vi "average_column_of_rand_matrix.vi"() -> ()   [LabVIEW 2021]
uses:
  <vilib>/Analysis/Matrix/Datatypes/RealMatrix.ctl
  <vilib>/Analysis/Matrix/Numeric/Conversions/Array To Matrix - RA2.vi
  <vilib>/Analysis/Matrix/NI_Matrix.lvlib
panel:
  out "sink array":dbl[][](array[numeric])
  out "sink mat":T1
  out "output":dbl[][](array[numeric])
  in  "loops":dbl
  in  "col index":dbl
  in  "blank":dbl[](array[numeric])
  out "avg":dbl
  out "num":dbl
  out "sum":dbl
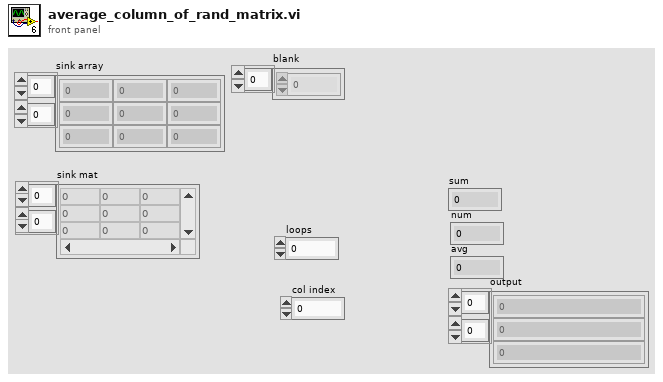
[diagram p1: front panel]
types:
  T1 = typedef "NI_Matrix.lvlib/RealMatrix.ctl" = dbl[][]
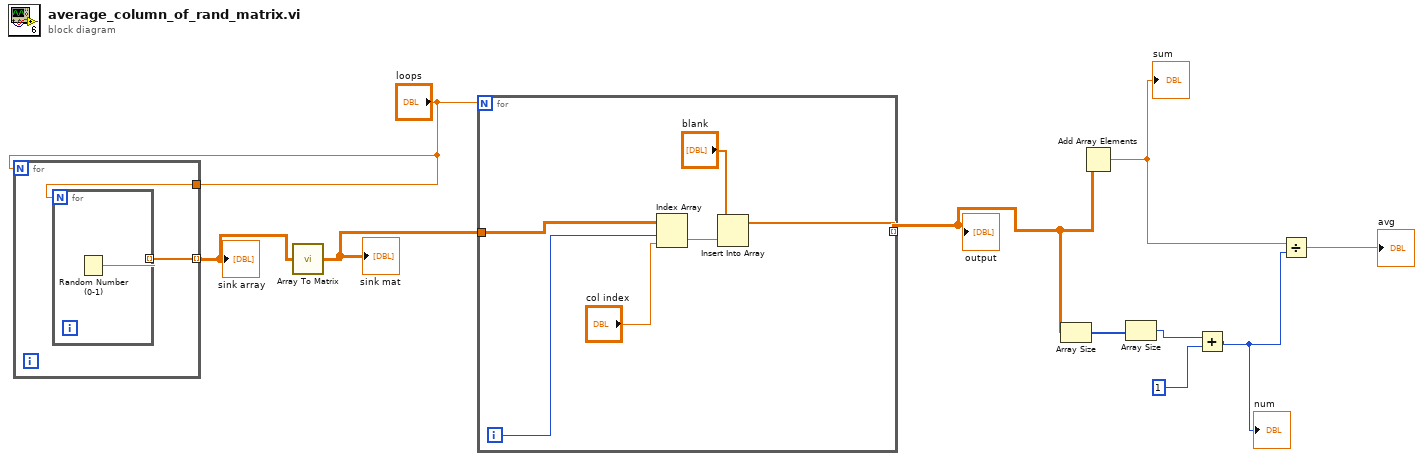
[diagram p0: block diagram]
diagram:
  n1 = for {
    N: "loops" -> [_]
    tunnel: [w12] -> w2 mode=indexing
    tunnel: "loops" -> [w11]
    n2 = for {
      N: w11 -> [_]
      tunnel: [w13] -> w12 mode=indexing
      n3 = Random Number (0-1)() -> (number: 0 to 1=w13:dbl)
    }
  }
  "sink array" <- w2
  n4 = call-poly <vilib>:"Array To Matrix.vi"("Real 2D Array"=w2) -> ("Real Matrix"=w1:T1)
  "sink mat" <- w1
  n5 = for {
    N: "loops" -> [_]
    tunnel: [w15] -> w8 mode=indexing
    tunnel: w1 -> [w14]
    i -> [w16]
    n6 = Index Array(array=w14, index (row)=w16, index (col)="col index") -> (element=w18:dbl)
    n7 = Insert Into Array(array="blank", new element=w18) -> (w15:dbl[])  [unwired: 1 in]
  }
  "output" <- w8
  n8 = Array Size(array=w8) -> (size(s)=w7:i32[])
  n9 = Add Array Elements(numeric array=w8) -> (sum=w10:dbl)
  "sum" <- w10
  n10 = Array Size(array=w7) -> (size(s)=w5:i32)
  n11 = Add(x=w5, y=1) -> (x+y=w4:i32)
  "num" <- w4
  n12 = Divide(x=w10, y=w4) -> (x/y=→"avg":dbl)
